vi "player_new-test.vi"() -> ()   [LabVIEW 2010]
uses:
  musicplayer_glo.vi
  player_glo.vi
panel:
  in  "playstate-array":dbl[](array[numeric])
  in  "loop-time":dbl=100.0
  in  "stop-all":bool
  out "error-pool":errorcluster caption="Fehler (Ausgang)"
  out "playerkernel referenz":refnum<vi>
  in  "position":ext(slide) scale=-1.0..337.789365
  in  "forward":bool
  out "playState":i32(ring) items=["wmppsUndefined", "wmppsStopped", "wmppsPaused", "wmppsPlaying", "wmppsScanForward", "wmppsScanReverse", "wmppsBuffering", "wmppsWaiting", "wmppsMediaEnded", "wmppsTransitioning", "wmppsReady", "wmppsReconnecting", "wmppsLast"]
  in  "pause":bool
  in  "stop":bool
  in  "start":bool
  in  "path":path
  in  "balance":i64(slide) scale=-100.0..100.0
  in  "volume":dbl(slide)=23.46938775510204 scale=0.0..100.0
  out "zeitmax":ext
  out "zeit":ext
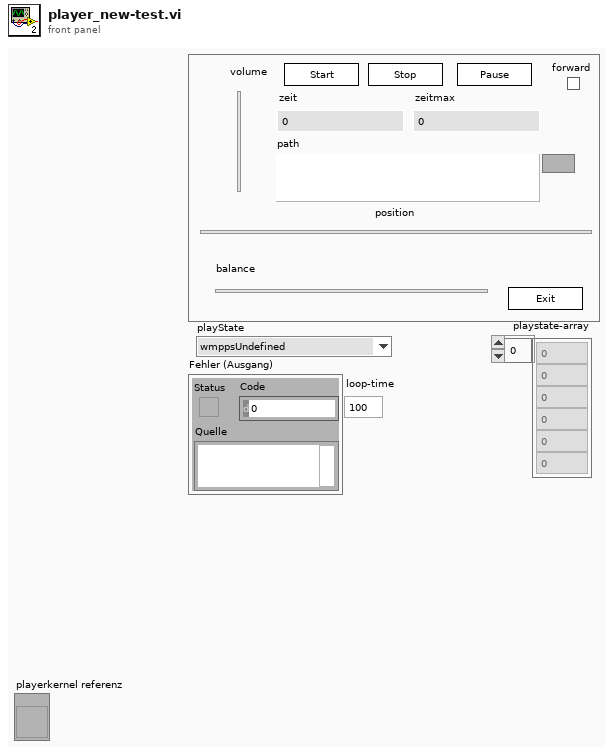
[diagram p1: front panel]
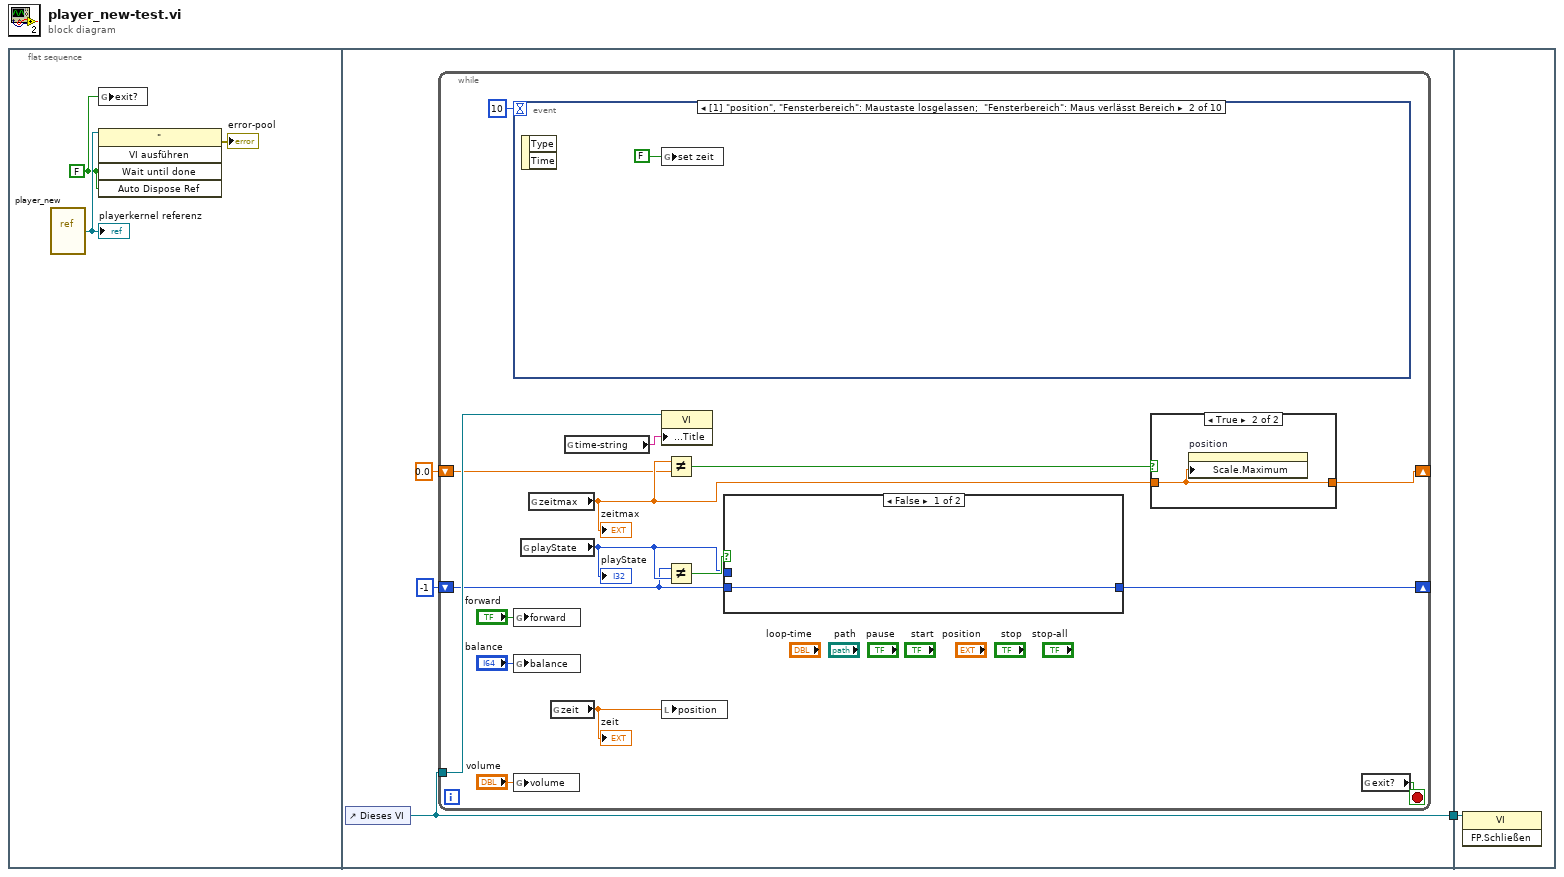
[diagram p0: block diagram]
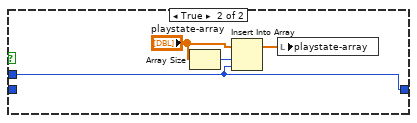
[diagram p2: hidden frame]
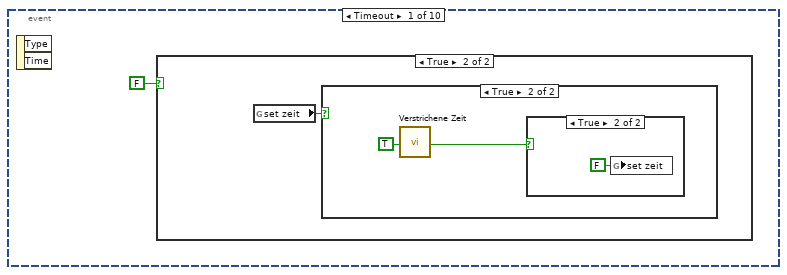
[diagram p4: hidden frame]
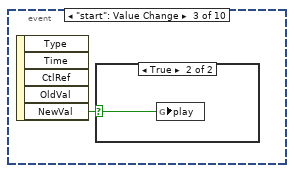
[diagram p8: hidden frame]
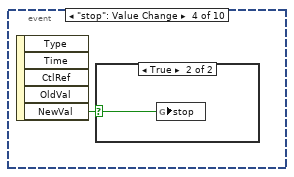
[diagram p10: hidden frame]
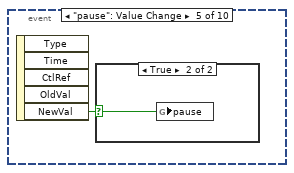
[diagram p12: hidden frame]
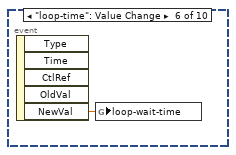
[diagram p14: hidden frame]
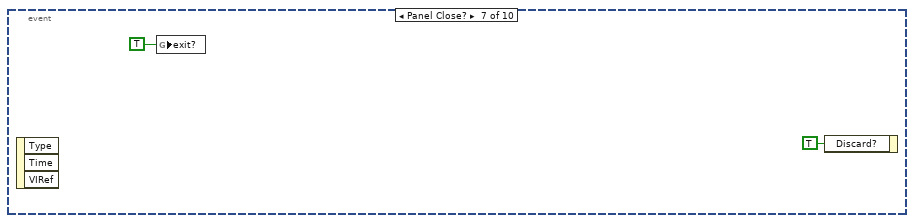
[diagram p15: hidden frame]
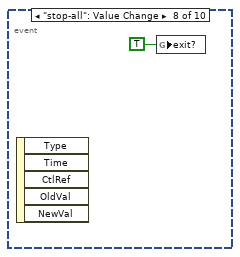
[diagram p16: hidden frame]
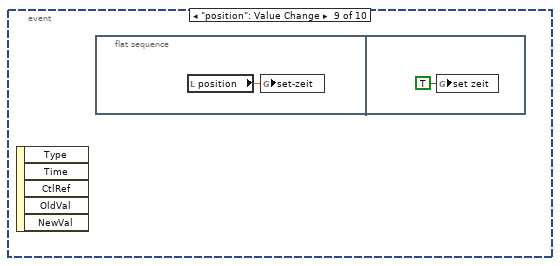
[diagram p17: hidden frame]
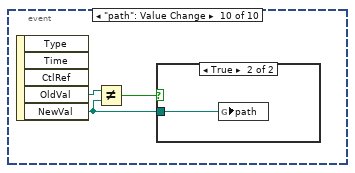
[diagram p18: hidden frame]
diagram:
  n1 = flat-sequence {
    tunnel: [w7] -> w1
    tunnel: w1 -> [w53]
    frame #0 {
      w2 = FALSE ("Warten bis beendet")
      n2 = vi-ref "player_new.vi"() -> (w4:refnum<vi>)
      "playerkernel referenz" <- w4
      n3 = global write "musicplayer_glo.vi" "exit?"(w2) -> ()
      n4 = invoke class="\"" method="VI ausführen"(reference=w4, "Wait until done"=w2, "Auto Dispose Ref"=w2) -> (error out=→"error-pool":errorcluster)  [unwired: 2 in, 4 out]
    }
    frame #1 {
      n5 = control-ref of="Dieses VI"() -> (w7:refnum<vi>)
      n6 = while {
        tunnel: w7 -> [w21]
        shift-right: [w16] -> _
        shift-left: 0.0 ("zeitmax") -> [w14]
        shift-right: [w9] -> _
        shift-left: -1 -> [w8]
        stop <- w17 stop-if-true
        n7 = event shown="[1] \"position\", \"Fensterbereich\": Maustaste losgelassen;  \"Fensterbereich\": Maus verlässt Bereich" {
          selector: _ -> [_ _ _ _ _ _ _ _ _ _]
          dyn-events: _ -> [_ _ _ _ _ _ _ _ _ _]
          timeout: 10 -> [_ _ _ _ _ _ _ _ _ _]
          event Timeout {
            n8 = event-data() -> ()  [unwired: 1 in, 2 out]
            n9 = case shown="True" FALSE {
              frame False {
              }
              frame True {
                n10 = global read "player_glo.vi" "set zeit"() -> (w32:bool)
                n11 = case shown="True" w32 {
                  frame False {
                  }
                  frame True {
                    n12 = call "Verstrichene Zeit"("Auto Reset"=TRUE) -> ("Time has Elapsed"=w34:bool)  [unwired: 11 in, 7 out]
                    n13 = case shown="True" w34 {
                      frame False {
                      }
                      frame True {
                        n14 = global write "player_glo.vi" "set zeit"(FALSE) -> ()
                      }
                    }
                  }
                }
              }
            }
          }
          event "position": Mouse Up; Mouse Leave {
            n15 = event-data() -> ()  [unwired: 1 in, 2 out]
            n16 = global write "player_glo.vi" "set zeit"(FALSE) -> ()
          }
          event "start": Value Change {
            n17 = event-data() -> ("NewVal"=w37:bool)  [unwired: 1 in, 4 out]
            n18 = case shown="True" w37 {
              selector: w37 -> [_ w38]
              frame False {
              }
              frame True {
                n19 = global write "player_glo.vi" "play"(w38) -> ()
              }
            }
          }
          event "stop": Value Change {
            n20 = event-data() -> ("NewVal"=w39:bool)  [unwired: 1 in, 4 out]
            n21 = case shown="True" w39 {
              selector: w39 -> [_ w40]
              frame False {
              }
              frame True {
                n22 = global write "player_glo.vi" "stop"(w40) -> ()
              }
            }
          }
          event "pause": Value Change {
            n23 = event-data() -> ("NewVal"=w41:bool)  [unwired: 1 in, 4 out]
            n24 = case shown="True" w41 {
              selector: w41 -> [_ w42]
              frame False {
              }
              frame True {
                n25 = global write "player_glo.vi" "pause"(w42) -> ()
              }
            }
          }
          event "loop-time": Value Change {
            n26 = event-data() -> ("NewVal"=w43:dbl)  [unwired: 1 in, 4 out]
            n27 = global write "player_glo.vi" "loop-wait-time"(w43) -> ()
          }
          event Panel Close? {
            n28 = event-data() -> ()  [unwired: 1 in, 3 out]
            n29 = global write "musicplayer_glo.vi" "exit?"(TRUE) -> ()
            n30 = event-data("Discard?"=TRUE ("Verwerfen?")) -> ()  [unwired: 1 in, 1 out]
          }
          event "stop-all": Value Change {
            n31 = event-data() -> ()  [unwired: 1 in, 5 out]
            n32 = global write "musicplayer_glo.vi" "exit?"(TRUE) -> ()
          }
          event "position": Value Change {
            n33 = event-data() -> ()  [unwired: 1 in, 5 out]
            n34 = flat-sequence {
              frame #0 {
                n35 = local read "position"() -> (w47:ext)
                n36 = global write "player_glo.vi" "set-zeit"(w47) -> ()
              }
              frame #1 {
                n37 = global write "player_glo.vi" "set zeit"(TRUE) -> ()
              }
            }
          }
          event "path": Value Change {
            n38 = event-data() -> ("OldVal"=w51:path, "NewVal"=w49:path)  [unwired: 1 in, 3 out]
            n39 = Not Equal?(x=w51, y=w49) -> (x != y?=w50:bool)
            n40 = case shown="True" w50 {
              tunnel: w49 -> [_ w52]
              frame False {
              }
              frame True {
                n41 = global write "player_glo.vi" "path"(w52) -> ()
              }
            }
          }
        }
        n42 = global write "player_glo.vi" "forward"("forward") -> ()
        n43 = global write "player_glo.vi" "balance"("balance") -> ()
        n44 = global write "player_glo.vi" "volume"("volume") -> ()
        n45 = global read "player_glo.vi" "playState"() -> (w10:i32)
        "playState" <- w10
        n46 = global read "player_glo.vi" "zeitmax"() -> (w15:dbl)
        "zeitmax" <- w15
        n47 = global read "player_glo.vi" "zeit"() -> (w18:dbl)
        "zeit" <- w18
        n48 = global read "player_glo.vi" "time-string"() -> (w22:string)
        n49 = property class="VI"(reference=w21, "Front Panel.Title"=w22) -> ()  [unwired: 1 in, 2 out]
        n50 = local write "position"(w18) -> ()
        n51 = Not Equal?(x=w15, y=w14) -> (x != y?=w13:bool)
        n52 = Not Equal?(x=w8, y=w10) -> (x != y?=w11:bool)
        n53 = case shown="False" w11 {
          tunnel: w10 -> [_ w25]
          tunnel: [w24 w25] -> w9
          tunnel: w8 -> [w24 _]
          frame False {
          }
          frame True {
            n54 = Array Size(array="playstate-array") -> (size(s)=w27:i32)
            n55 = Insert Into Array(array="playstate-array", index=w27, new element=w25) -> (w26:dbl[])
            n56 = local write "playstate-array"(w26) -> ()
          }
        }
        n57 = case shown="True" w13 {
          tunnel: w15 -> [w29 w30]
          tunnel: [w29 w30] -> w16
          frame False {
          }
          frame True {
            n58 = property on="position" class="Schieber (strikt)"("Scale.Maximum"=w30) -> ()  [unwired: 2 in, 2 out]
          }
        }
        n59 = global read "musicplayer_glo.vi" "exit?"() -> (w17:bool)
      }
    }
    frame #2 {
      n60 = invoke class="VI" method="FP.Schließen"(reference=w53) -> ()  [unwired: 2 in, 3 out]
    }
  }
